vi "Write Last of Header Contents Class Array.vi"(8 "error in (no error)":errorcluster, 10 "Simulated_Header.lvclass":refnum<class "Simulated_Header.lvclass">, 11 "Save Image in":refnum<class "Save Image.lvclass">) -> (0 "error out":errorcluster, 3 "Save Image out":refnum<class "Save Image.lvclass">)   [LabVIEW 2018, in "Save Image.lvclass"]
uses:
  Save Image.lvclass
  Simulated_Header/Simulated_Header.lvclass
  Save Image.lvclass/Save Image.ctl
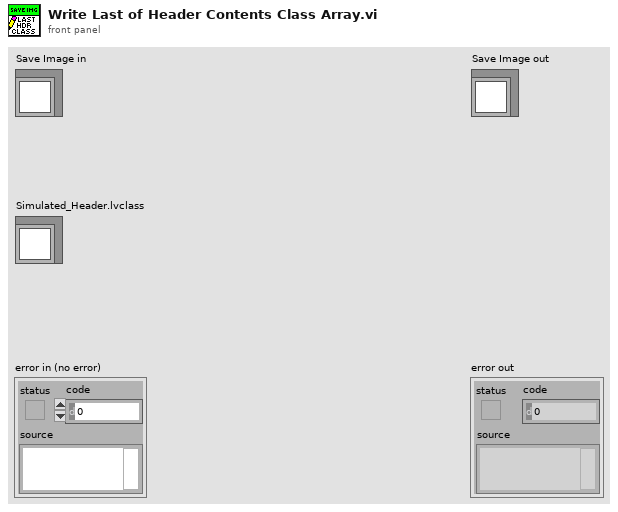
[diagram p1: front panel]
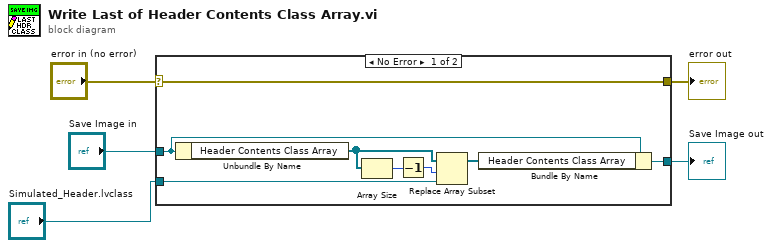
[diagram p0: block diagram]
diagram:
  n1 = case shown="No Error" "error in (no error)" {
    selector: "error in (no error)" -> [w13 w14]
    tunnel: [w13 w14] -> w4
    tunnel: [w12 w15] -> w2
    tunnel: "Save Image in" -> [w11 w15]
    tunnel: "Simulated_Header.lvclass" -> [w9 _]
    frame No Error {
      n2 = Unbundle By Name(w11) -> ("Header Contents Class Array"=w8:refnum<class "Simulated_Header.lvclass">[])
      n3 = Array Size(array=w8) -> (size(s)=w7:i32)
      n4 = Decrement(x=w7) -> (x-1=w6:i32)
      n5 = Replace Array Subset(array=w8, new element=w9, index=w6) -> (w10:refnum<class "Simulated_Header.lvclass">[])
      n6 = Bundle By Name(cluster=w11, "Header Contents Class Array"=w10) -> (w12:refnum<class "Save Image.lvclass">)
    }
    frame Error {
    }
  }
  "error out" <- w4
  "Save Image out" <- w2
